vi "scan2d_DO_perform_scan.vi"(8 "error in (no error)":errorcluster, 10 "scan-2d-settings":T1, 11 "scan_panel in":refnum<class "scan_2d.lvclass">) -> (0 "error out":errorcluster, 3 "scan_panel out":refnum<class "scan_2d.lvclass">)   [LabVIEW 2015, in "scan_2d.lvclass"]
uses:
  scan_2d.lvclass
  scan_2d_settings.ctl
  Scan/scan_record.ctl
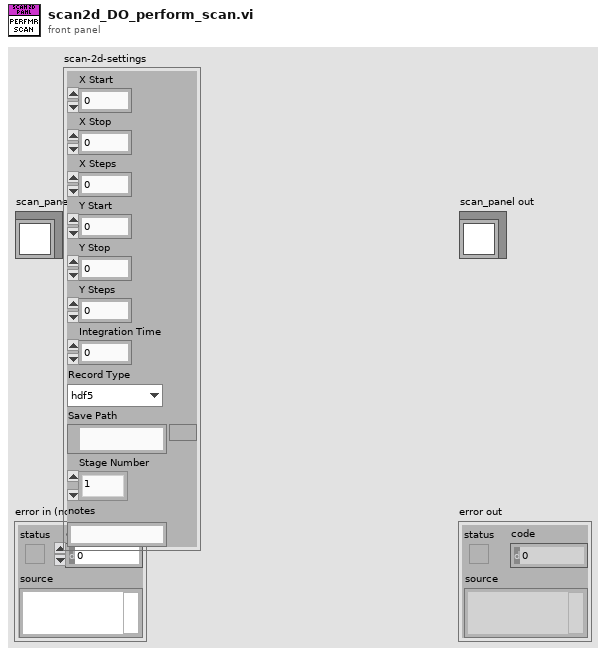
[diagram p1: front panel]
types:
  T1 = typedef "scan_2d_settings.ctl" = cluster{"X Start":dbl, "X Stop":dbl, "X Steps":u32, "Y Start":dbl, "Y Stop":dbl, "Y Steps":u32, "Integration Time":dbl, "Record Type":T2, "Save Path":path, "Stage Number":enum16{"1", "2"}, "notes":string}
  T2 = typedef "scan_record.ctl" = enum16{"hdf5", "legacy", "None"}
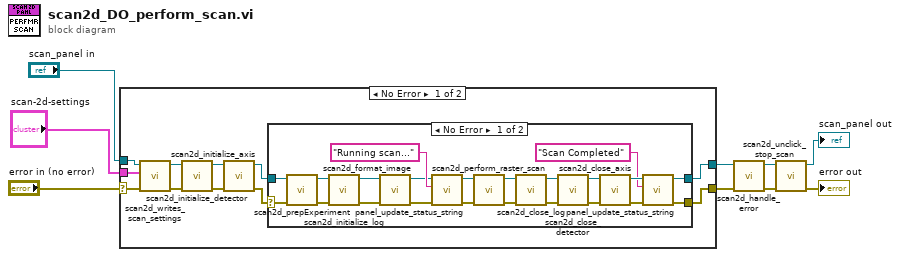
[diagram p0: block diagram]
diagram:
  n1 = case shown="No Error" "error in (no error)" {
    selector: "error in (no error)" -> [w12 w46]
    tunnel: "scan_panel in" -> [w20 w45]
    tunnel: "scan-2d-settings" -> [w17 _]
    tunnel: [w10 w46] -> w4
    tunnel: [w11 w45] -> w2
    frame No Error {
      n2 = call "scan2d_writes_scan_settings.vi"("error in (no error)"=w12, "scan-2d-settings"=w17, "scan_2d in"=w20) -> ("error out"=w18:errorcluster, "scan_2d out"=w19:refnum<class "scan_2d.lvclass">)  [unwired: 7 in]
      n3 = call "scan2d_initialize_detector.vi"("error in (no error)"=w18, "scan_2d in"=w19) -> ("error out"=w16:errorcluster, "scan_2d out"=w15:refnum<class "scan_2d.lvclass">)  [unwired: 8 in]
      n4 = call "scan2d_initialize_axis.vi"("error in (no error)"=w16, "scan_2d in"=w15) -> ("error out"=w13:errorcluster, "scan_2d out"=w14:refnum<class "scan_2d.lvclass">)  [unwired: 8 in]
      n5 = case shown="No Error" w13 {
        selector: w13 -> [w21 w43]
        tunnel: w14 -> [w42 w44]
        tunnel: [w24 w43] -> w10
        tunnel: [w23 w44] -> w11
        frame No Error {
          n6 = call "scan2d_prepExperiment.vi"("error in (no error)"=w21, "scan_2d in"=w42) -> ("error out"=w41:errorcluster, "scan_2d out"=w40:refnum<class "scan_2d.lvclass">)  [unwired: 8 in]
          n7 = call "scan2d_initialize_log.vi"("error in (no error)"=w41, "scan_2d in"=w40) -> ("error out"=w39:errorcluster, "scan_2d out"=w38:refnum<class "scan_2d.lvclass">)  [unwired: 8 in]
          n8 = call "scan2d_format_image.vi"("error in (no error)"=w39, "scan_panel in"=w38) -> ("error out"=w36:errorcluster, "panel out"=w35:refnum<class "scan_2d.lvclass">)  [unwired: 8 in]
          n9 = call-dynamic "panel_update_status_string.vi"("error in (no error)"=w36, "String"="Running scan...", "scan_panel in"=w35) -> ("error out"=w34:errorcluster, "scan_panel out"=w33:refnum<class "scan_2d.lvclass">)  [unwired: 7 in]
          n10 = call "scan2d_perform_raster_scan.vi"("error in (no error)"=w34, "scan_2d in"=w33) -> ("error out"=w32:errorcluster, "scan_2d out"=w31:refnum<class "scan_2d.lvclass">)  [unwired: 8 in]
          n11 = call "scan2d_close_log.vi"("error in (no error)"=w32, "scan_2d in"=w31) -> ("error out"=w29:errorcluster, "scan_2d out"=w30:refnum<class "scan_2d.lvclass">)  [unwired: 8 in]
          n12 = call "scan2d_close_detector.vi"("error in (no error)"=w29, "scan_2d in"=w30) -> ("error out"=w28:errorcluster, "scan_2d out"=w27:refnum<class "scan_2d.lvclass">)  [unwired: 8 in]
          n13 = call "scan2d_close_axis.vi"("error in (no error)"=w28, "scan_2d in"=w27) -> ("error out"=w25:errorcluster, "scan_2d out"=w26:refnum<class "scan_2d.lvclass">)  [unwired: 8 in]
          n14 = call-dynamic "panel_update_status_string.vi"("error in (no error)"=w25, "String"="Scan Completed", "scan_panel in"=w26) -> ("error out"=w24:errorcluster, "scan_panel out"=w23:refnum<class "scan_2d.lvclass">)  [unwired: 7 in]
        }
        frame Error {
        }
      }
    }
    frame Error {
    }
  }
  n15 = call "scan2d_handle_error.vi"("error in (no error)"=w4, "scan_panel in"=w2) -> ("error out"=w3:errorcluster, "scan_panel out"=w1:refnum<class "scan_2d.lvclass">)  [unwired: 8 in]
  n16 = call "scan2d_unclick_stop_scan.vi"("error in (no error)"=w3, "scan_panel in"=w1) -> ("error out"=→"error out":errorcluster, "scan_panel out"=→"scan_panel out":refnum<class "scan_2d.lvclass">)  [unwired: 8 in]
